vi "Create Data Updated Observer.vi"(8 "error in (no error)":errorcluster) -> (0 "error out":errorcluster, 3 "Main Controller":refnum<event-registration>)   [LabVIEW 2015, in "Main Controller Actor.lvclass"]
uses:
  Main Controller Actor.lvclass
  Re-use Libraries/Minimal Actor Framework/Actors/Base Actor/Actor/Update User Event.ctl
  Re-use Libraries/Minimal Actor Framework/Actors/Base Actor/Actor/Actor.lvclass
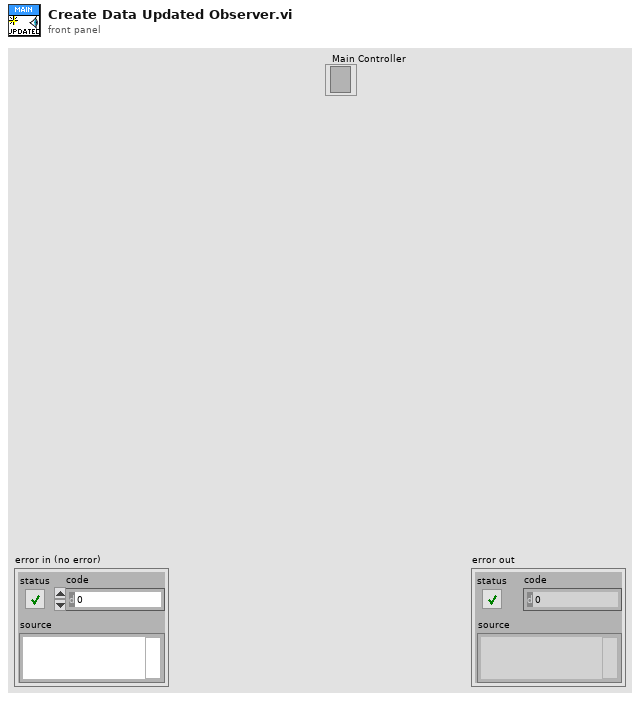
[diagram p1: front panel]
types:
  T1 = typedef "Actor.lvclass/Update User Event.ctl" = refnum<user-event>
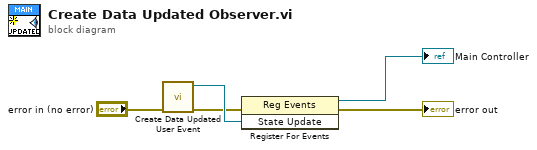
[diagram p0: block diagram]
diagram:
  n1 = call "Create Data Updated User Event.vi"("error in (no error)"="error in (no error)") -> ("error out"=w3:errorcluster, "State Update"=w4:T1)  [unwired: 9 in]
  n2 = register-events(error in=w3, w4) -> (reference out=→"Main Controller":refnum<event-registration>, error out=→"error out":errorcluster)  [unwired: 1 in]
